vi "Measure IV DC.vi"(0 "dI or Imin":dbl=1e-06, 1 "Imax":dbl=1e-05, 2 "IV Sampling":enum16{"Linear", "Logartihmic"}(ring)=enum."Logartihmic", 3 "IV Type":T1(ring), 4 "6221 Address":string="12", 5 "Ipts":i32=31, 6 "Period (s)":string="0.5", 8 "2182A Address":string="8", 9 "2182A Buffer":string="11") -> (7 "Data array":dbl[][](array[numeric])=[[3e-06, 4.3047886363637716e-07, 1.5313515229084694e-08, 0.14349295454545904, 0.005104505076361564], [3.141e-06, 4.451970222646495e-07, 1.6482457125202314e-08, 0.14173735188304665, 0.005247518982872433], [3.288e-06, 4.509710933322839e-07, 2.1111679012790933e-08, 0.13715665855604742, 0.006420826950362206], [3.442e-06, 4.68688173379921e-07, 1.7706994792785522e-08, 0.136167394938966, 0.005144391282041116], [3.603e-06, 4.984350637099025e-07, 1.7680289772848306e-08, 0.13833890194557383, 0.004907102351609299], [3.772e-06, 5.251681368726084e-07, 2.1467663960858997e-08, 0.1392280320447, 0.005691321304575556], [3.949e-06, 5.275954224918868e-07, 1.1682564654597293e-08, 0.13360228475357985, 0.002958360256925119], [4.134e-06, 5.748183520129533e-07, 1.682018898207155e-08, 0.13904652927260602, 0.004068744311096166], [4.328e-06, 6.067757953443141e-07, 2.4132014421245018e-08, 0.1401977345989635, 0.005575788914335725], [4.531e-06, 6.208427140441133e-07, 2.1984855414698184e-08, 0.13702112426486718, 0.004852097862436147], [4.744e-06, 6.53840833567312e-07, 1.8213175774497554e-08, 0.1378247962831602, 0.0038392023133426547], [4.966e-06, 6.972885085498247e-07, 1.2757960522883814e-08, 0.14041250675590508, 0.0025690617243020165], [5.199e-06, 7.373899562843383e-07, 1.8464251029463237e-08, 0.1418330364078358, 0.003551500486528801], [5.443e-06, 7.869491881659043e-07, 2.1658645151036676e-08, 0.14458004559358886, 0.0039791741964057825], [5.698e-06, 8.296971125303819e-07, 2.6760166214436293e-08, 0.14561198886107088, 0.004696413867047436], [5.965e-06, 8.769758274541976e-07, 1.618644186342838e-08, 0.147020256069438, 0.0027135694657884966], [6.245e-06, 9.014262408876311e-07, 1.6360553186388587e-08, 0.14434367348080562, 0.0026197843372920073], [6.537e-06, 9.540709106298745e-07, 6.51123628419529e-09, 0.1459493514807824, 0.0009960587860173306], [6.844e-06, 9.83842449902655e-07, 2.1788031573785793e-08, 0.14375254966432716, 0.0031835230236390696], [7.165e-06, 1.0389678276192175e-06, 1.6974003144092472e-08, 0.14500597733694592, 0.00236901648905687], [7.501e-06, 1.0842385707281058e-06, 1.7358394306252265e-08, 0.1445458699810833, 0.002314144021630751], [7.852e-06, 1.133576332443823e-06, 2.5546159944328773e-08, 0.14436784671979405, 0.0032534589842497163], [8.221e-06, 1.1828825836341094e-06, 2.5139338002287402e-08, 0.14388548639266627, 0.0030579416132207036], [8.606e-06, 1.2298374260108544e-06, 2.3631436253352804e-08, 0.14290465094246507, 0.002745925662718197], [9.009e-06, 1.316429879745037e-06, 2.1479730496761806e-08, 0.14612386277556189, 0.00238425246939303], [9.432e-06, 1.3727473526086722e-06, 1.6611977521761823e-08, 0.14554149200685668, 0.0017612359543852654], [9.874e-06, 1.440120416246957e-06, 1.667890150606247e-08, 0.1458497484552316, 0.0016891737397268045], [1.0337e-05, 1.4833079536573893e-06, 2.558120171970024e-08, 0.14349501341369733, 0.002474722039247387], [1.0822e-05, 1.552698820767039e-06, 1.7381109531494778e-08, 0.14347614311282933, 0.0016060903281736071], [1.1329e-05, 1.625415578548681e-06, 1.746370239359197e-08, 0.14347387929637928, 0.0015415043157906232], [1.186e-05, 1.7084207500312594e-06, 2.1510520309515023e-08, 0.1440489671189932, 0.0018137032301446057], [1.2416e-05, 1.7752295908882855e-06, 1.866622301771358e-08, 0.14297918741046114, 0.001503400694081313], [1.2998e-05, 1.8543913473684005e-06, 2.184911828979089e-08, 0.14266743709558397, 0.0016809600161402439], [1.3608e-05, 1.9194233726401615e-06, 2.432538101843289e-08, 0.1410511002821988, 0.0017875794399201124], [1.4246e-05, 2.004528849673536e-06, 1.642871958280506e-08, 0.14070818824045597, 0.001153216312144115], [1.4914e-05, 2.1149393689095325e-06, 2.049443802084905e-08, 0.14180899617202175, 0.0013741744683417629], [1.5613e-05, 2.2048839061364533e-06, 2.6366973762175795e-08, 0.1412210277420389, 0.0016887833063585342], [1.6345e-05, 2.299442544196895e-06, 2.4227330364434726e-08, 0.1406817096480205, 0.0014822471926849022], [1.7111e-05, 2.415440098271509e-06, 2.4366737884075522e-08, 0.1411630003080772, 0.001424039383091317], [1.7914e-05, 2.524075530215886e-06, 2.826235852574557e-08, 0.14089960534865947, 0.001577668780046085], [1.8753e-05, 2.649793418562226e-06, 1.806602988302559e-08, 0.14129970770341949, 0.0009633674549685698], [1.9633e-05, 2.777555497862733e-06, 1.9031456611346844e-08, 0.14147381948060575, 0.0009693605975320554], [2.0553e-05, 2.9073259128042663e-06, 1.884648667183435e-08, 0.14145506314427414, 0.0009169701100488663], [2.1517e-05, 3.01009900374514e-06, 1.7512218724119184e-08, 0.13989399097202862, 0.0008138782694668952], [2.2526e-05, 3.160053215899305e-06, 2.1388694840911432e-08, 0.14028470282781252, 0.0009495114463691481], [2.3582e-05, 3.2978086632925506e-06, 2.184497068877449e-08, 0.13984431614335302, 0.0009263408824007502], [2.4687e-05, 3.4422688886650723e-06, 1.9324922599488052e-08, 0.13943650053327955, 0.0007827975290431423], [2.5845e-05, 3.600770279715974e-06, 2.1454878390334967e-08, 0.13932173649510443, 0.000830136521196942], [2.7056e-05, 3.78881652021074e-06, 2.6607076592041645e-08, 0.14003609255657673, 0.0009834076209358975], [2.8325e-05, 3.959486400941646e-06, 2.0862877075484172e-08, 0.13978769288408283, 0.0007365534713321861], [2.9653e-05, 4.17532703440116e-06, 2.3495754463244276e-08, 0.14080622649988736, 0.0007923567417544356], [3.1043e-05, 4.363664112839576e-06, 2.1355539918027872e-08, 0.14056837653704785, 0.00068793415320774], [3.2499e-05, 4.565058439581727e-06, 2.8015991032708503e-08, 0.14046765868432035, 0.0008620570181454353], [3.4023e-05, 4.7549412581003e-06, 2.443505404219635e-08, 0.13975667219528848, 0.0007181922241482629], [3.5618e-05, 4.987050296574805e-06, 1.9740604892462154e-08, 0.1400148884433378, 0.0005542311441535784], [3.7288e-05, 5.248996848807335e-06, 3.229313460677829e-08, 0.14076906374188303, 0.0008660463046228892], [3.9036e-05, 5.512797242351469e-06, 2.5164798391517365e-08, 0.14122341536918406, 0.0006446561735709951], [4.0866e-05, 5.775482443930134e-06, 2.5641849608176923e-08, 0.1413273245223446, 0.0006274616945181061], [4.2782e-05, 6.0405987288507725e-06, 1.9151097766145253e-08, 0.1411948653370757, 0.00044764381670200676], [4.4788e-05, 6.3309968379260555e-06, 2.226396665998493e-08, 0.1413547565849347, 0.0004970966924172754], [4.6888e-05, 6.625184069244457e-06, 3.3556500197253995e-08, 0.14129807347817047, 0.0007156735240840726], [4.9086e-05, 6.952019006582743e-06, 2.894434069415916e-08, 0.14162936492243702, 0.0005896659066568709], [5.1387e-05, 7.288042561715788e-06, 3.348238378409694e-08, 0.14182658185369426, 0.0006515730395644217], [5.3797e-05, 7.650843163495064e-06, 4.295870622361934e-08, 0.14221691104513381, 0.0007985334911541413], [5.6319e-05, 8.029530359919404e-06, 3.787768783183094e-08, 0.14257231768886883, 0.0006725561148427873], [5.896e-05, 8.411537190961149e-06, 3.588480477149981e-08, 0.14266514910042655, 0.0006086296603035924], [6.1724e-05, 8.816997123246386e-06, 4.1323845634023504e-08, 0.14284552399790013, 0.0006694939672416484], [6.4618e-05, 9.252996924901479e-06, 2.9598595842858586e-08, 0.14319534688324428, 0.0004580549667717755], [6.7647e-05, 9.726133083514764e-06, 6.354616463109044e-08, 0.14377774451956132, 0.0009393789027021219], [7.0819e-05, 1.0171226654104171e-05, 2.4735429811748093e-08, 0.14362285056417304, 0.0003492767451072183], [7.4139e-05, 1.0733877514461845e-05, 2.553373296049051e-08, 0.14478044638397936, 0.00034440352527671683], [7.7615e-05, 1.1272707367916842e-05, 3.785521497216293e-08, 0.14523877301960758, 0.0004877306573750297], [8.1254e-05, 1.1873621776794473e-05, 5.281513040074092e-08, 0.14612968932968803, 0.0006500003741445457], [8.5064e-05, 1.2483718740590531e-05, 5.2611155735638645e-08, 0.1467567800784178, 0.0006184890874593088], [8.9052e-05, 1.3137543120825948e-05, 5.422691673347627e-08, 0.14752664870891108, 0.00060893541676185], [9.3227e-05, 1.386324379852252e-05, 5.440153662832007e-08, 0.1487041715224401, 0.000583538423721884], [9.7598e-05, 1.4592835245281601e-05, 4.026019591612147e-08, 0.14951981849301832, 0.0004125104604205155], [0.000102174, 1.5381084091995798e-05, 5.398714968184118e-08, 0.1505381417189872, 0.000528384419537663], [0.000106965, 1.6288471088931045e-05, 5.8580991496088557e-08, 0.15227851249409663, 0.0005476650446042028], [0.00011198, 1.7226805678510595e-05, 4.938284161551474e-08, 0.1538382361002911, 0.0004409969781703406], [0.00011723, 1.8195690188901986e-05, 8.422935795560593e-08, 0.1552135988134606, 0.0007184966131161472], [0.000122726, 1.9440666602087193e-05, 4.754013298598356e-07, 0.1584070743125922, 0.003873680637027489], [0.00012848, 2.046516097520856e-05, 7.72151635638954e-08, 0.15928674482572044, 0.0006009897537663093], [0.000134504, 2.1783101356090124e-05, 6.206822937093433e-08, 0.16195132751509342, 0.00046146010059875043], [0.00014081, 2.3186551308853717e-05, 6.909433376080896e-08, 0.16466551600634696, 0.0004906919519977911], [0.000147412, 2.4779199580014395e-05, 1.0145495447783537e-07, 0.1680948605270561, 0.000688240811316822], [0.000154324, 2.652754000838863e-05, 1.1552426768280052e-07, 0.17189510386193094, 0.0007485826422513706], [0.000161559, 2.8559074860751355e-05, 1.5325269701068354e-07, 0.17677179767608958, 0.000948586565964654], [0.000169134, 3.077335985603851e-05, 1.0749987858342273e-07, 0.1819466213537107, 0.0006355899971822503], [0.000177064, 3.3499875105511105e-05, 1.650934863194129e-07, 0.1891964210992133, 0.0009323944241596987], [0.000185365, 3.675271060014896e-05, 2.140875156213152e-07, 0.19827211501712275, 0.0011549511268109686], [0.000194056, 4.0755061588877246e-05, 2.4656490232316033e-07, 0.21001701358822839, 0.0012705863375683326], [0.000203154, 4.5583701866592996e-05, 2.88002297844996e-07, 0.22438003616267954, 0.0014176550687901592], [0.000212679, 4.6885277578993986e-05, 1.8559705682216518e-07, 0.22045090290528913, 0.0008726628243604925], [0.000222651, 5.437543406576834e-05, 3.339108756556848e-07, 0.24421823421304345, 0.0014997052591530459], [0.00023309, 6.52378590218662e-05, 4.087905596822482e-07, 0.27988270205442617, 0.001753788492351659], [0.000244018, 8.078607685365366e-05, 5.535103789648243e-07, 0.33106605600264594, 0.0022683178247704036], [0.000255459, 0.00010528381597780848, 7.381396785359974e-07, 0.4121358651596087, 0.0028894643701572365], [0.000267436, 0.00014543789662409701, 1.3105807197850573e-06, 0.5438231824589697, 0.004900539642325855], [0.000279975, 0.0002164796371265307, 1.9276740217917436e-06, 0.7732105978267013, 0.006885164824687003], [0.000293101, 0.0003364904621252049, 1.684747078560466e-06, 1.1480358720209243, 0.005748008633749002], [0.000306843, 0.0005085274541554971, 1.1729721508444118e-06, 1.6572887572976966, 0.003822711128637159], [0.00032123, 0.0006778030568942108, 6.876202556105575e-07, 2.1100241474775423, 0.002140585423561179], [0.000336291, 0.0008259884419767413, 4.1136515560515926e-07, 2.456171714309159, 0.0012232416437108315], [0.000352057, 0.0009578186150472369, 1.982003546971834e-07, 2.7206350535488197, 0.0005629780254253811], [0.000368564, 0.0010792919557635811, 2.0647815388337988e-07, 2.928370529307206, 0.000560223336743089], [0.000385844, 0.0011932501573751963, 1.6637910902181772e-07, 3.092571498779808, 0.00043120823188080604], [0.000403934, 0.0013019248018429324, 6.616749526058568e-08, 3.2231126912885086, 0.00016380768952498596], [0.000422872, 0.0014063865904152633, 5.9536173907995785e-08, 3.3257973817497097, 0.00014079005918574836], [0.000442699, 0.0015057233089116322, 5.663047245823841e-08, 3.40123494498888, 0.00012792094054479096], [0.000463455, 0.001602269073650902, 2.8720907727946024e-08, 3.457226858380861, 6.197129759727703e-05], [0.000485184, 0.0016952998337987934, 2.339000992951633e-08, 3.494137963739104, 4.820853517328752e-05], [0.000507932, 0.001786953980172823, 1.5693892498723275e-08, 3.5180968715749805, 3.089762507328397e-05], [0.000531746, 0.001878406864318594, 1.5599137248114433e-08, 3.5325265527499856, 2.9335692695599837e-05], [0.000556677, 0.0019710559814260058, 1.0823648816328349e-08, 3.5407534017500377, 1.94433195844778e-05], [0.000582777, 0.002065715042834221, 1.3096483346757564e-08, 3.5446063294093983, 2.2472546697549086e-05], [0.0006101, 0.002163659391303364, 1.0976700998578674e-08, 3.546401231442983, 1.7991642351382843e-05], [0.000638705, 0.0022654655576607543, 1.1177311405105967e-08, 3.5469669998837556, 1.749995914405863e-05], [0.00066865, 0.0023721142447375295, 1.5030529513429894e-08, 3.5476172059186863, 2.2478919484677922e-05], [0.0007, 0.002483311050336363, 1.5199603028809162e-08, 3.547587214766233, 2.1713718612584518e-05]])   [LabVIEW 2020]
uses:
  <vilib>/Analysis/1siggen.llb/Ramp Pattern by Delta.vi
  <vilib>/Analysis/NI_AALBase.lvlib
panel:
  in  "Correct Voltage Offset":bool=TRUE
  out "Voltage Offset":dbl=2.1003043299999988e-05
  in  "Debug Mode":bool
  out "Resistance STD":dbl=2.1713718612584518e-05
  out "Resistance":dbl=3.5475872147662333
  in  "NPLC":string="1"
  in  "2182A Range":string="0.01"
  out "I-V Plot":cluster{"Ramp Pattern":dbl[], dbl[]}[](graph)=[{"Ramp Pattern"=[3e-06, 3.141e-06, 3.288e-06, 3.442e-06, 3.603e-06, 3.772e-06, 3.949e-06, 4.134e-06, 4.328e-06, 4.531e-06, 4.744e-06, 4.966e-06, 5.199e-06, 5.443e-06, 5.698e-06, 5.965e-06, 6.245e-06, 6.537e-06, 6.844e-06, 7.165e-06, 7.501e-06, 7.852e-06, 8.221e-06, 8.606e-06, 9.009e-06, 9.432e-06, 9.874e-06, 1.0337e-05, 1.0822e-05, 1.1329e-05, 1.186e-05, 1.2416e-05, 1.2998e-05, 1.3608e-05, 1.4246e-05, 1.4914e-05, 1.5613e-05, 1.6345e-05, 1.7111e-05, 1.7914e-05, 1.8753e-05, 1.9633e-05, 2.0553e-05, 2.1517e-05, 2.2526e-05, 2.3582e-05, 2.4687e-05, 2.5845e-05, 2.7056e-05, 2.8325e-05, 2.9653e-05, 3.1043e-05, 3.2499e-05, 3.4023e-05, 3.5618e-05, 3.7288e-05, 3.9036e-05, 4.0866e-05, 4.2782e-05, 4.4788e-05, 4.6888e-05, 4.9086e-05, 5.1387e-05, 5.3797e-05, 5.6319e-05, 5.896e-05, 6.1724e-05, 6.4618e-05, 6.7647e-05, 7.0819e-05, 7.4139e-05, 7.7615e-05, 8.1254e-05, 8.5064e-05, 8.9052e-05, 9.3227e-05, 9.7598e-05, 0.000102174, 0.000106965, 0.00011198, 0.00011723, 0.000122726, 0.00012848, 0.000134504, 0.00014081, 0.000147412, 0.000154324, 0.000161559, 0.000169134, 0.000177064, 0.000185365, 0.000194056, 0.000203154, 0.000212679, 0.000222651, 0.00023309, 0.000244018, 0.000255459, 0.000267436, 0.000279975, 0.000293101, 0.000306843, 0.00032123, 0.000336291, 0.000352057, 0.000368564, 0.000385844, 0.000403934, 0.000422872, 0.000442699, 0.000463455, 0.000485184, 0.000507932, 0.000531746, 0.000556677, 0.000582777, 0.0006101, 0.000638705, 0.00066865, 0.0007], [4.3047886363637716e-07, 4.451970222646495e-07, 4.509710933322839e-07, 4.68688173379921e-07, 4.984350637099025e-07, 5.251681368726084e-07, 5.275954224918868e-07, 5.748183520129533e-07, 6.067757953443141e-07, 6.208427140441133e-07, 6.53840833567312e-07, 6.972885085498247e-07, 7.373899562843383e-07, 7.869491881659043e-07, 8.296971125303819e-07, 8.769758274541976e-07, 9.014262408876311e-07, 9.540709106298745e-07, 9.83842449902655e-07, 1.0389678276192175e-06, 1.0842385707281058e-06, 1.133576332443823e-06, 1.1828825836341094e-06, 1.2298374260108544e-06, 1.316429879745037e-06, 1.3727473526086722e-06, 1.440120416246957e-06, 1.4833079536573893e-06, 1.552698820767039e-06, 1.625415578548681e-06, 1.7084207500312594e-06, 1.7752295908882855e-06, 1.8543913473684005e-06, 1.9194233726401615e-06, 2.004528849673536e-06, 2.1149393689095325e-06, 2.2048839061364533e-06, 2.299442544196895e-06, 2.415440098271509e-06, 2.524075530215886e-06, 2.649793418562226e-06, 2.777555497862733e-06, 2.9073259128042663e-06, 3.01009900374514e-06, 3.160053215899305e-06, 3.2978086632925506e-06, 3.4422688886650723e-06, 3.600770279715974e-06, 3.78881652021074e-06, 3.959486400941646e-06, 4.17532703440116e-06, 4.363664112839576e-06, 4.565058439581727e-06, 4.7549412581003e-06, 4.987050296574805e-06, 5.248996848807335e-06, 5.512797242351469e-06, 5.775482443930134e-06, 6.0405987288507725e-06, 6.3309968379260555e-06, 6.625184069244457e-06, 6.952019006582743e-06, 7.288042561715788e-06, 7.650843163495064e-06, 8.029530359919404e-06, 8.411537190961149e-06, 8.816997123246386e-06, 9.252996924901479e-06, 9.726133083514764e-06, 1.0171226654104171e-05, 1.0733877514461845e-05, 1.1272707367916842e-05, 1.1873621776794473e-05, 1.2483718740590531e-05, 1.3137543120825948e-05, 1.386324379852252e-05, 1.4592835245281601e-05, 1.5381084091995798e-05, 1.6288471088931045e-05, 1.7226805678510595e-05, 1.8195690188901986e-05, 1.9440666602087193e-05, 2.046516097520856e-05, 2.1783101356090124e-05, 2.3186551308853717e-05, 2.4779199580014395e-05, 2.652754000838863e-05, 2.8559074860751355e-05, 3.077335985603851e-05, 3.3499875105511105e-05, 3.675271060014896e-05, 4.0755061588877246e-05, 4.5583701866592996e-05, 4.6885277578993986e-05, 5.437543406576834e-05, 6.52378590218662e-05, 8.078607685365366e-05, 0.00010528381597780848, 0.00014543789662409701, 0.0002164796371265307, 0.0003364904621252049, 0.0005085274541554971, 0.0006778030568942108, 0.0008259884419767413, 0.0009578186150472369, 0.0010792919557635811, 0.0011932501573751963, 0.0013019248018429324, 0.0014063865904152633, 0.0015057233089116322, 0.001602269073650902, 0.0016952998337987934, 0.001786953980172823, 0.001878406864318594, 0.0019710559814260058, 0.002065715042834221, 0.002163659391303364, 0.0022654655576607543, 0.0023721142447375295, 0.002483311050336363]}, {"Ramp Pattern"=[3e-06, 3.141e-06, 3.288e-06, 3.442e-06, 3.603e-06, 3.772e-06, 3.949e-06, 4.134e-06, 4.328e-06, 4.531e-06, 4.744e-06, 4.966e-06, 5.199e-06, 5.443e-06, 5.698e-06, 5.965e-06, 6.245e-06, 6.537e-06, 6.844e-06, 7.165e-06, 7.501e-06, 7.852e-06, 8.221e-06, 8.606e-06, 9.009e-06, 9.432e-06, 9.874e-06, 1.0337e-05, 1.0822e-05, 1.1329e-05, 1.186e-05, 1.2416e-05, 1.2998e-05, 1.3608e-05, 1.4246e-05, 1.4914e-05, 1.5613e-05, 1.6345e-05, 1.7111e-05, 1.7914e-05, 1.8753e-05, 1.9633e-05, 2.0553e-05, 2.1517e-05, 2.2526e-05, 2.3582e-05, 2.4687e-05, 2.5845e-05, 2.7056e-05, 2.8325e-05, 2.9653e-05, 3.1043e-05, 3.2499e-05, 3.4023e-05, 3.5618e-05, 3.7288e-05, 3.9036e-05, 4.0866e-05, 4.2782e-05, 4.4788e-05, 4.6888e-05, 4.9086e-05, 5.1387e-05, 5.3797e-05, 5.6319e-05, 5.896e-05, 6.1724e-05, 6.4618e-05, 6.7647e-05, 7.0819e-05, 7.4139e-05, 7.7615e-05, 8.1254e-05, 8.5064e-05, 8.9052e-05, 9.3227e-05, 9.7598e-05, 0.000102174, 0.000106965, 0.00011198, 0.00011723, 0.000122726, 0.00012848, 0.000134504, 0.00014081, 0.000147412, 0.000154324, 0.000161559, 0.000169134, 0.000177064, 0.000185365, 0.000194056, 0.000203154, 0.000212679, 0.000222651, 0.00023309, 0.000244018, 0.000255459, 0.000267436, 0.000279975, 0.000293101, 0.000306843, 0.00032123, 0.000336291, 0.000352057, 0.000368564, 0.000385844, 0.000403934, 0.000422872, 0.000442699, 0.000463455, 0.000485184, 0.000507932, 0.000531746, 0.000556677, 0.000582777, 0.0006101, 0.000638705, 0.00066865, 0.0007], [0.14349295454545904, 0.14173735188304665, 0.13715665855604742, 0.136167394938966, 0.13833890194557383, 0.1392280320447, 0.13360228475357985, 0.13904652927260602, 0.1401977345989635, 0.13702112426486718, 0.1378247962831602, 0.14041250675590508, 0.1418330364078358, 0.14458004559358886, 0.14561198886107088, 0.147020256069438, 0.14434367348080562, 0.1459493514807824, 0.14375254966432716, 0.14500597733694592, 0.1445458699810833, 0.14436784671979405, 0.14388548639266627, 0.14290465094246507, 0.14612386277556189, 0.14554149200685668, 0.1458497484552316, 0.14349501341369733, 0.14347614311282933, 0.14347387929637928, 0.1440489671189932, 0.14297918741046114, 0.14266743709558397, 0.1410511002821988, 0.14070818824045597, 0.14180899617202175, 0.1412210277420389, 0.1406817096480205, 0.1411630003080772, 0.14089960534865947, 0.14129970770341949, 0.14147381948060575, 0.14145506314427414, 0.13989399097202862, 0.14028470282781252, 0.13984431614335302, 0.13943650053327955, 0.13932173649510443, 0.14003609255657673, 0.13978769288408283, 0.14080622649988736, 0.14056837653704785, 0.14046765868432035, 0.13975667219528848, 0.1400148884433378, 0.14076906374188303, 0.14122341536918406, 0.1413273245223446, 0.1411948653370757, 0.1413547565849347, 0.14129807347817047, 0.14162936492243702, 0.14182658185369426, 0.14221691104513381, 0.14257231768886883, 0.14266514910042655, 0.14284552399790013, 0.14319534688324428, 0.14377774451956132, 0.14362285056417304, 0.14478044638397936, 0.14523877301960758, 0.14612968932968803, 0.1467567800784178, 0.14752664870891108, 0.1487041715224401, 0.14951981849301832, 0.1505381417189872, 0.15227851249409663, 0.1538382361002911, 0.1552135988134606, 0.1584070743125922, 0.15928674482572044, 0.16195132751509342, 0.16466551600634696, 0.1680948605270561, 0.17189510386193094, 0.17677179767608958, 0.1819466213537107, 0.1891964210992133, 0.19827211501712275, 0.21001701358822839, 0.22438003616267954, 0.22045090290528913, 0.24421823421304345, 0.27988270205442617, 0.33106605600264594, 0.4121358651596087, 0.5438231824589697, 0.7732105978267013, 1.1480358720209243, 1.6572887572976966, 2.1100241474775423, 2.456171714309159, 2.7206350535488197, 2.928370529307206, 3.092571498779808, 3.2231126912885086, 3.3257973817497097, 3.40123494498888, 3.457226858380861, 3.494137963739104, 3.5180968715749805, 3.5325265527499856, 3.5407534017500377, 3.5446063294093983, 3.546401231442983, 3.5469669998837556, 3.5476172059186863, 3.547587214766233]}]
  out "Votlage STD":dbl=1.5199603028809162e-08
  out "Voltage":dbl=0.002483311050336363
  out "Current Now":string="700.000E-6"
  in  "stop":bool
  in  "Measure?":bool=TRUE
  out "Current Samples":dbl[](array[numeric])=[3e-06, 3.1406549088857057e-06, 3.2879044189026255e-06, 3.442057717724511e-06, 3.603438489279804e-06, 3.772385593408102e-06, 3.9492537773822905e-06, 4.134414420790367e-06, 4.32825631534104e-06, 4.531186481230464e-06, 4.743631021784333e-06, 4.966036018169827e-06, 5.198868466056096e-06, 5.442617256190057e-06, 5.697794200946451e-06, 5.9649351090076585e-06, 6.244600910429864e-06, 6.537378834457898e-06, 6.8438836425619034e-06, 7.164758919284874e-06, 7.50067842361156e-06, 7.852347503696246e-06, 8.220504577920009e-06, 8.605922685387296e-06, 9.009411109117489e-06, 9.431817075339749e-06, 9.874027532459264e-06, 1.0336971013430267e-05, 1.0821619585446334e-05, 1.1328990891041906e-05, 1.1860150284890736e-05, 1.2416213070788092e-05, 1.2998346843513827e-05, 1.3607773940493573e-05, 1.4245774008406035e-05, 1.4913686690125602e-05, 1.5612914437642126e-05, 1.6344925456864413e-05, 1.711125679049072e-05, 1.791351754541951e-05, 1.875339227147733e-05, 1.9632644498558175e-05, 2.0553120439601558e-05, 2.151675286718458e-05, 2.2525565171867943e-05, 2.358167561081731e-05, 2.468730175562123e-05, 2.5844765148644834e-05, 2.7056496177696535e-05, 2.8325039179243306e-05, 2.9653057780890138e-05, 3.1043340494341355e-05, 3.249880657058786e-05, 3.402251212961459e-05, 3.561765657749918e-05, 3.728758932437601e-05, 3.9035816817371893e-05, 4.0866009903280735e-05, 4.2782011536436836e-05, 4.4787844847971736e-05, 4.688772159339793e-05, 4.908605099625717e-05, 5.138744900640303e-05, 5.379674799235784e-05, 5.631900688809529e-05, 5.895952181555477e-05, 6.172383720519199e-05, 6.461775743791608e-05, 6.764735903285898e-05, 7.081900340656744e-05, 7.413935023040985e-05, 7.761537141424442e-05, 8.125436574571134e-05, 8.506397421588756e-05, 8.905219606348478e-05, 9.32274055712786e-05, 9.759836965003821e-05, 0.00010217426624687807, 0.0001069647036166842, 0.00011197974049708122, 0.00011722990722930185, 0.00012272622786930757, 0.00012848024333558884, 0.000134504035642249, 0.00014081025326825573, 0.0001474121377161289, 0.00015432355131583193, 0.00016155900633224755, 0.00016913369543735668, 0.00017706352361110468, 0.00018536514153793865, 0.0001940559805691401, 0.00020315428932436634, 0.00021267917200925264, 0.00022265062852953554, 0.0002330895964859245, 0.00024401799513790236, 0.00025545877142876697, 0.0002674359481685561, 0.0002799746744760263, 0.00029310127858560314, 0.0003068433231301837, 0.0003212296630158713, 0.00033629050601016584, 0.0003520574761708282, 0.0003685636802486078, 0.00038584377720325734, 0.00040393405097880397, 0.0004228724866908901, 0.00044269885038614946, 0.0004634547725411065, 0.0004851838354759112, 0.0005079316648664714, 0.0005317460255471244, 0.000556676921805013, 0.0005827767023767664, 0.0006101001703679381, 0.0006387046983260229, 0.0006686503487086629, 0.0006999999999999999]
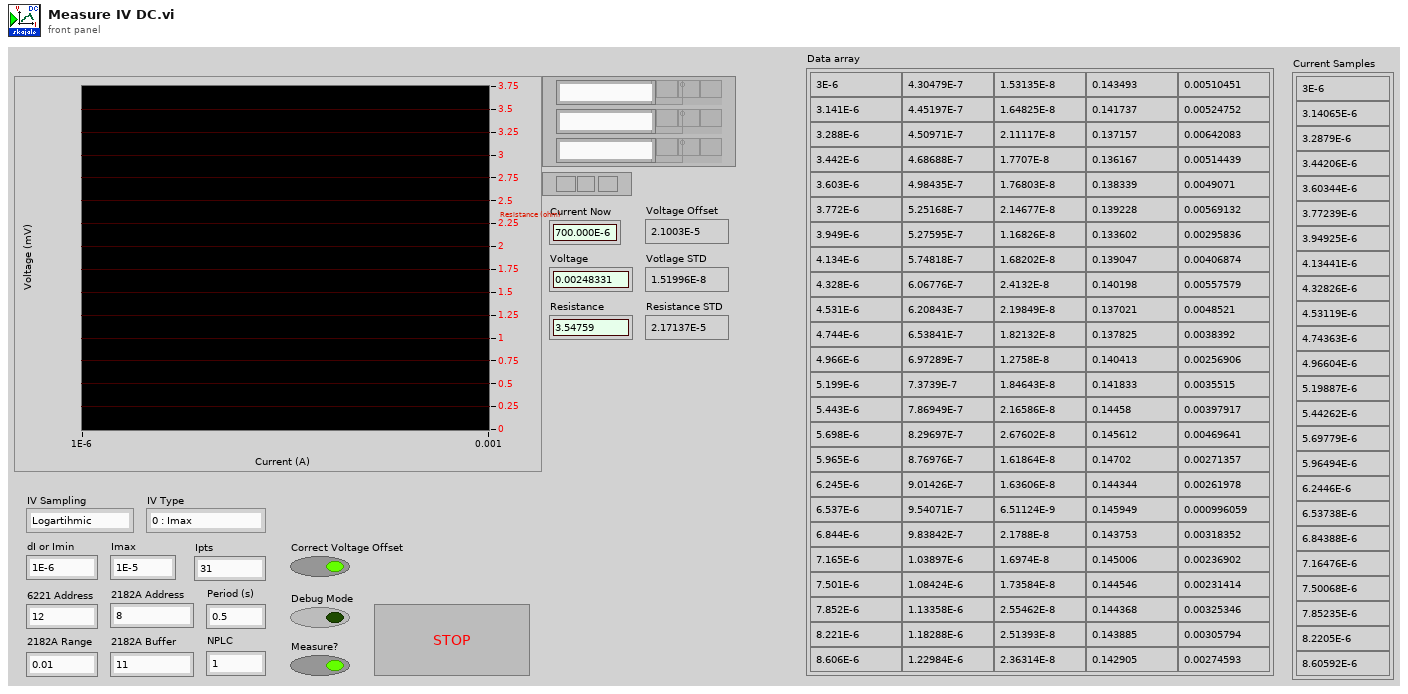
[diagram p1: front panel]
types:
  T1 = enum16{"0 : Imax", "0 : Imax : 0", "0 : Imax : -Imax : 0", "-Imax : 0 : Imax"}
  T2 = cluster{"Data array":dbl[], "Data array":dbl[]}[]
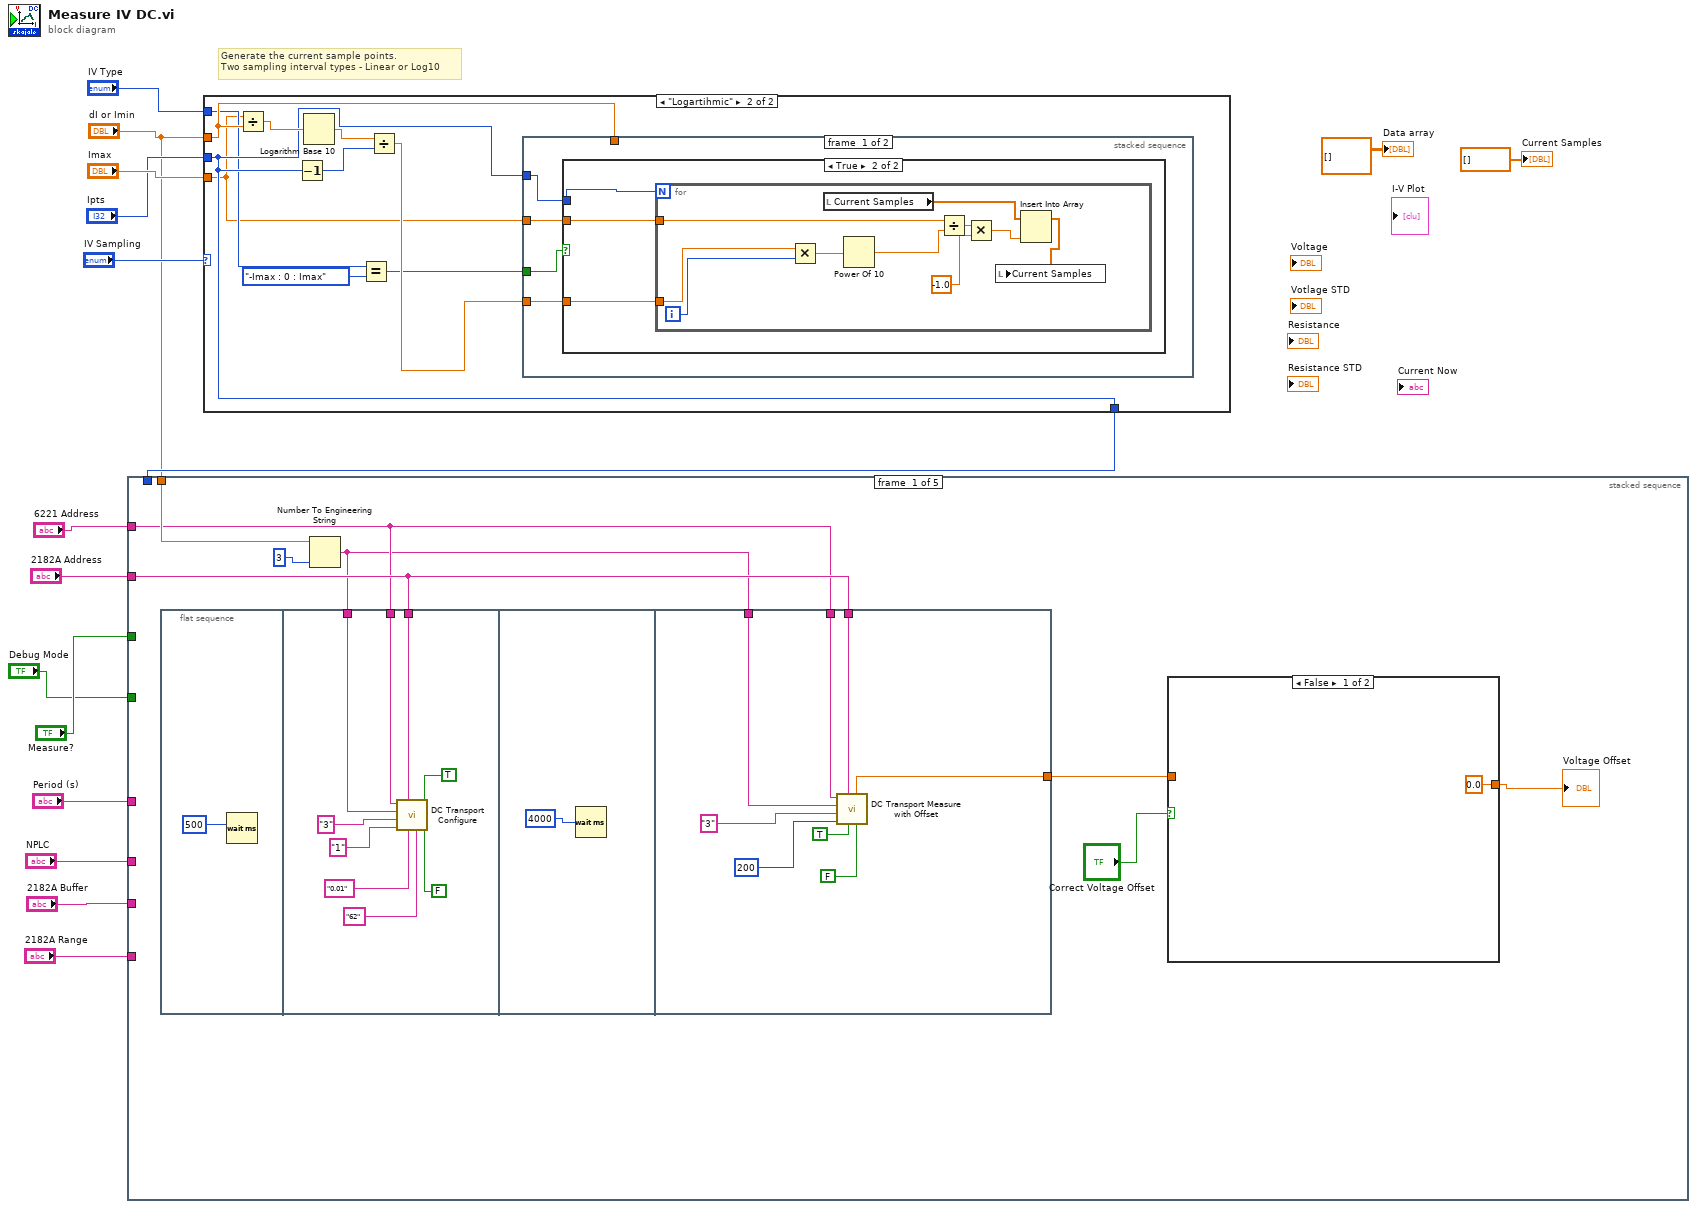
[diagram p0: block diagram]
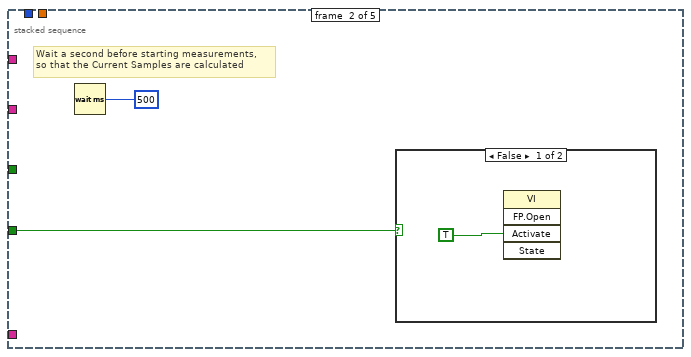
[diagram p3: hidden frame]
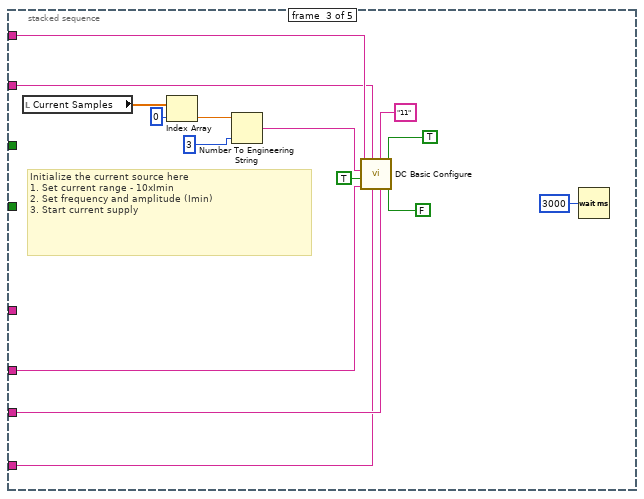
[diagram p5: hidden frame]
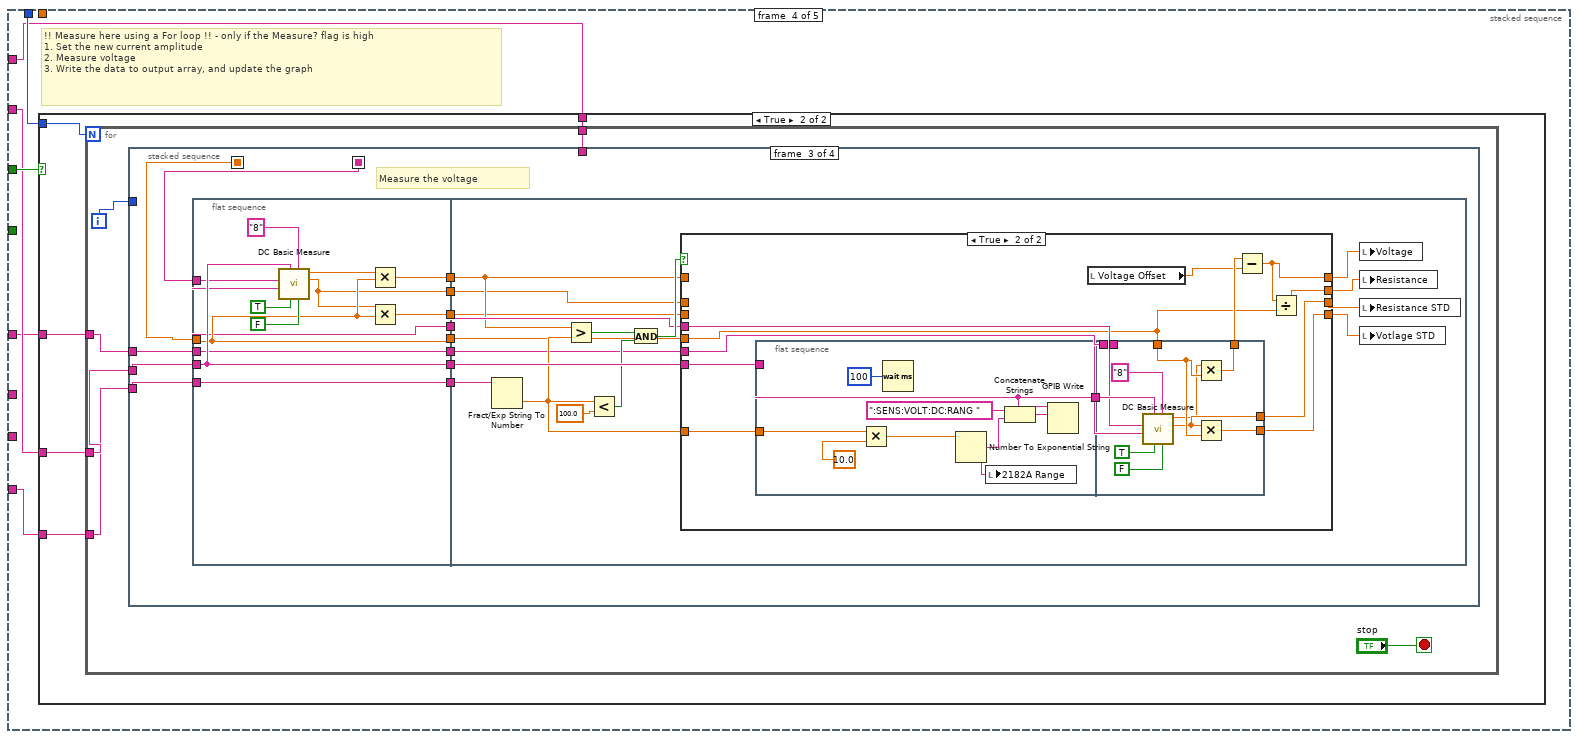
[diagram p6: hidden frame]
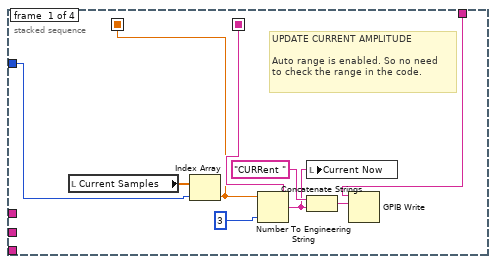
[diagram p8: hidden frame]
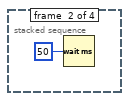
[diagram p9: hidden frame]
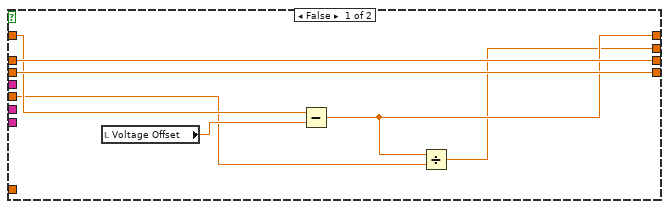
[diagram p10: hidden frame]
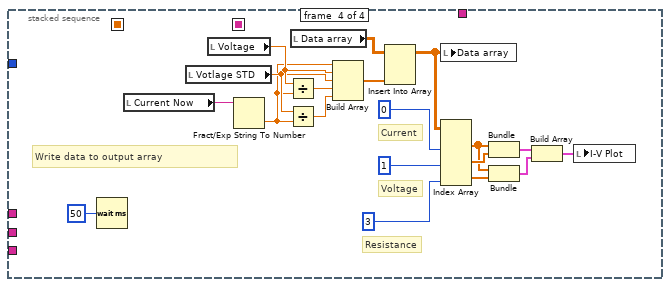
[diagram p11: hidden frame]
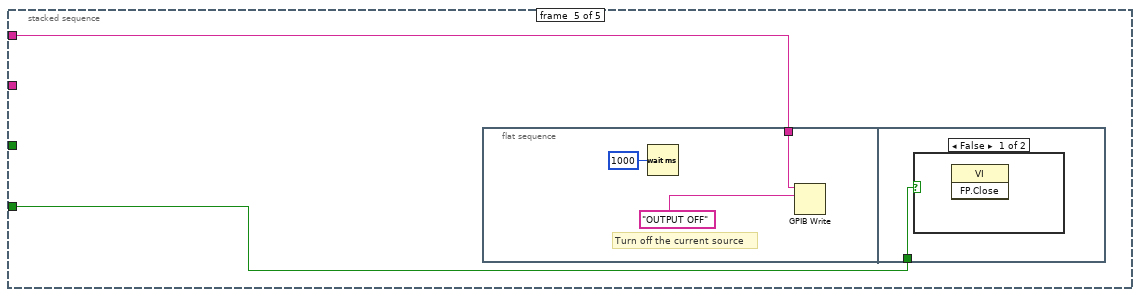
[diagram p12: hidden frame]
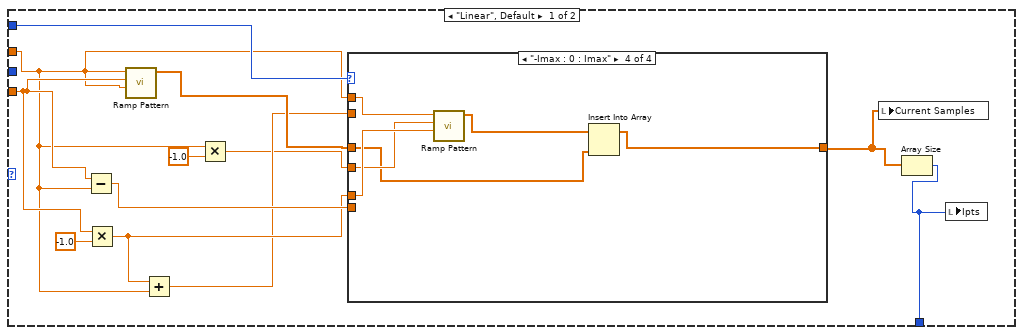
[diagram p14: hidden frame]
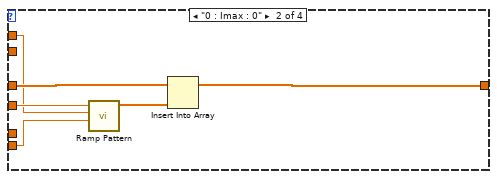
[diagram p16: hidden frame]
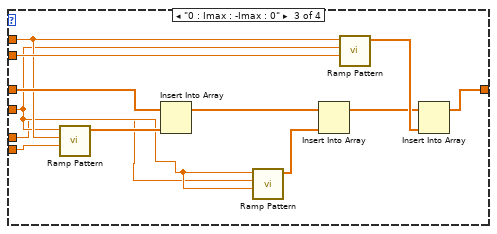
[diagram p17: hidden frame]
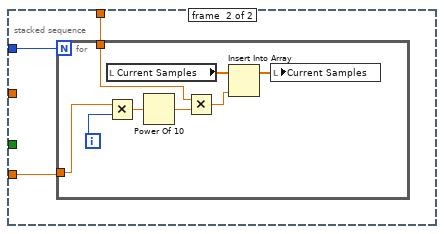
[diagram p19: hidden frame]
diagram:
  # "Generate the current sample points.\nTwo sampling interval types - Linear or Log10"
  n1 = case shown="\"Logartihmic\"" "IV Sampling" {
    tunnel: "Ipts" -> [_ w58]
    tunnel: "Imax" -> [w24 w54]
    tunnel: "dI or Imin" -> [w18 w59]
    tunnel: "IV Type" -> [w28 w57]
    tunnel: [w17 w58] -> w2
    frame "Linear", Default {
      n2 = Subtract(x=w24, y=w18) -> (x-y=w26:dbl)
      n3 = Multiply(x=w24, y=-1.0) -> (x*y=w23:dbl)
      n4 = call-poly <vilib>:"Ramp Pattern.vi"("start"=w18, "end"=w24, "delta"=w18) -> ("Ramp Pattern"=w27:dbl[])  [unwired: 6 in, 2 out]
      n5 = Add(x=w23, y=w18) -> (x+y=w22:dbl)
      n6 = Multiply(x=w18, y=-1.0) -> (x*y=w20:dbl)
      n7 = case shown="\"-Imax : 0 : Imax\"" w28 {
        tunnel: w27 -> [w29 w34 w46 w49]
        tunnel: [w29 w32 w44 w48] -> w19
        tunnel: w26 -> [_ w35 w47 _]
        tunnel: w18 -> [_ w30 w41 w53]
        tunnel: w23 -> [_ _ w39 w52]
        tunnel: w22 -> [_ _ w43 _]
        tunnel: w20 -> [_ w31 w40 w51]
        frame "0 : Imax", Default {
          # "For Linear sampling, possible to choose sweep type\n- Forward, 0:Imax\n-Half cycle, 0:Imax:0\n- Full cycles, 0:Imax:-Imax:0"
          # "Pass on the 0:Imax samples are they are"
        }
        frame "0 : Imax : 0" {
          n8 = call-poly <vilib>:"Ramp Pattern.vi"("start"=w35, "end"=w30, "delta"=w31) -> ("Ramp Pattern"=w33:dbl[])  [unwired: 6 in, 2 out]
          n9 = Insert Into Array(array=w34, new element=w33) -> (w32:dbl[])  [unwired: 1 in]
        }
        frame "0 : Imax : -Imax : 0" {
          n10 = call-poly <vilib>:"Ramp Pattern.vi"("start"=w47, "end"=w41, "delta"=w40) -> ("Ramp Pattern"=w45:dbl[])  [unwired: 6 in, 2 out]
          n11 = Insert Into Array(array=w46, new element=w45) -> (w38:dbl[])  [unwired: 1 in]
          n12 = call-poly <vilib>:"Ramp Pattern.vi"("start"=w40, "end"=w39, "delta"=w40) -> ("Ramp Pattern"=w36:dbl[])  [unwired: 6 in, 2 out]
          n13 = Insert Into Array(array=w38, new element=w36) -> (w37:dbl[])  [unwired: 1 in]
          n14 = call-poly <vilib>:"Ramp Pattern.vi"("start"=w43, "end"=w40, "delta"=w41) -> ("Ramp Pattern"=w42:dbl[])  [unwired: 6 in, 2 out]
          n15 = Insert Into Array(array=w37, new element=w42) -> (w44:dbl[])  [unwired: 1 in]
        }
        frame "-Imax : 0 : Imax" {
          n16 = call-poly <vilib>:"Ramp Pattern.vi"("start"=w52, "end"=w51, "delta"=w53) -> ("Ramp Pattern"=w50:dbl[])  [unwired: 6 in, 2 out]
          n17 = Insert Into Array(array=w50, new element=w49) -> (w48:dbl[])  [unwired: 1 in]
        }
      }
      n18 = local write "Current Samples"(w19) -> ()
      n19 = Array Size(array=w19) -> (size(s)=w17:i32)
      n20 = local write "Ipts"(w17) -> ()
    }
    frame "Logartihmic" {
      n21 = Divide(x=w54, y=w59) -> (x/y=w63:dbl)
      n22 = Decrement(x=w58) -> (x-1=w61:i32)
      n23 = Logarithm Base 10(1:w63) -> (0:w62:dbl)
      n24 = Equal?(x=w57, y=T1."-Imax : 0 : Imax") -> (x = y?=w55:bool)
      n25 = Divide(x=w62, y=w61) -> (x/y=w60:dbl)
      n26 = stacked-sequence {
        tunnel: w60 -> [w66 w82]
        tunnel: w58 -> [w67 w81]
        tunnel: w59 -> [_ w83]
        tunnel: w55 -> [w65 _]
        tunnel: w54 -> [w64 _]
        frame #0 {
          n27 = case shown="True" w65 {
            tunnel: w67 -> [_ w70]
            tunnel: w66 -> [_ w69]
            tunnel: w64 -> [_ w68]
            frame False {
            }
            frame True {
              n28 = for {
                N: w70 -> [_]
                tunnel: w69 -> [w74]
                tunnel: w68 -> [w71]
                i -> [w80]
                n29 = Multiply(x=w74, y=w80) -> (x*y=w79:dbl)
                n30 = local read "Current Samples"() -> (w72:dbl[])
                n31 = Power Of 10(x=w79) -> (10^x=w77:dbl)
                n32 = Divide(x=w71, y=w77) -> (x/y=w78:dbl)
                n33 = Multiply(x=w78, y=-1.0) -> (x*y=w76:dbl)
                n34 = Insert Into Array(array=w72, new element=w76) -> (w73:dbl[])  [unwired: 1 in]
                n35 = local write "Current Samples"(w73) -> ()
              }
            }
          }
        }
        frame #1 {
          n36 = for {
            N: w81 -> [_]
            tunnel: w82 -> [w89]
            tunnel: w83 -> [w85]
            i -> [w88]
            n37 = local read "Current Samples"() -> (w90:dbl[])
            n38 = Multiply(x=w89, y=w88) -> (x*y=w87:dbl)
            n39 = Power Of 10(x=w87) -> (10^x=w86:dbl)
            n40 = Multiply(x=w85, y=w86) -> (x*y=w84:dbl)
            n41 = Insert Into Array(array=w90, new element=w84) -> (w91:dbl[])  [unwired: 1 in]
            n42 = local write "Current Samples"(w91) -> ()
          }
        }
      }
    }
  }
  n43 = stacked-sequence {
    tunnel: w2 -> [_ _ _ w144 _]
    tunnel: "2182A Buffer" -> [_ _ w133 _ _]
    tunnel: "2182A Range" -> [_ _ w132 w140 _]
    tunnel: "NPLC" -> [_ _ w131 _ _]
    tunnel: "6221 Address" -> [w96 _ w129 w139 w264]
    tunnel: "2182A Address" -> [w97 _ w128 w142 _]
    tunnel: "Measure?" -> [_ _ _ w143 _]
    tunnel: "Period (s)" -> [_ _ _ w141 _]
    tunnel: "Debug Mode" -> [_ w121 _ _ w265]
    tunnel: "dI or Imin" -> [w98 _ _ _ _]
    frame #0 {
      n44 = flat-sequence {
        tunnel: w97 -> [w110]
        tunnel: w96 -> [w109]
        tunnel: w95 -> [w108]
        tunnel: w97 -> [w120]
        tunnel: w96 -> [w119]
        tunnel: w95 -> [w118]
        tunnel: [w113] -> w93
        frame #0 {
          n45 = Wait (ms)(milliseconds to wait=u32 500) -> ()  [unwired: 1 out]
        }
        frame #1 {
          n46 = call "DC Transport Configure.vi"("Channel 2"=FALSE, "Channel 1"=TRUE, "Voltmeter Buffer Size"="62", "Voltmeter Range (V)"="0.01", "Voltmeter 1 Address"=w110, "NPLC"="1", "Time Period (s)"="3", "Current Amplitude"=w108, "6221 Address"=w109) -> ()  [unwired: 3 in]
        }
        frame #2 {
          n47 = Wait (ms)(milliseconds to wait=u32 4000) -> ()  [unwired: 1 out]
        }
        frame #3 {
          n48 = call "DC Transport Measure with Offset.vi"("Channel 2"=FALSE, "Channel 1"=TRUE, "Voltmeter 1 Address"=w120, "tpad"=200, "Period (s)"="3", "Amplitude (A)"=w118, "6221 Address"=w119) -> ("Voltmeter 1 Offset"=w113:dbl)  [unwired: 4 out]
        }
      }
      n49 = Number To Engineering String(2:i16 3 ("precision (6)"), 4:w98) -> (0:w95:string)  [unwired: 2 in]
      n50 = case shown="False" "Correct Voltage Offset" {
        tunnel: w93 -> [_ w101]
        tunnel: [0.0 ("Voltmeter 1 Offset") w101] -> w92
        frame False {
        }
        frame True {
        }
      }
      "Voltage Offset" <- w92
    }
    frame #1 {
      # "Wait a second before starting measurements,\nso that the Current Samples are calculated"
      n51 = Wait (ms)(milliseconds to wait=u32 500) -> ()  [unwired: 1 out]
      n52 = case shown="False" w121 {
        frame False {
          n53 = invoke class="VI" method="FP.Open"("Activate"=TRUE ("Activate?")) -> ()  [unwired: 4 in, 5 out]
        }
        frame True {
        }
      }
    }
    frame #2 {
      # "Initialize the current source here\n1. Set current range - 10xImin\n2. Set frequency and amplitude (Imin)\n3. Start current supply"
      n54 = local read "Current Samples"() -> (w138:dbl[])
      n55 = Index Array(array=w138, index=0) -> (element=w136:dbl)
      n56 = Number To Engineering String(2:i16 3 ("precision (6)"), 4:w136) -> (0:w130:string)  [unwired: 2 in]
      n57 = call "DC Basic Configure.vi"("Channel 2"=FALSE, "Channel 1"=TRUE, "Voltmeter Buffer Size"=w133, "Voltmeter 2 Address"="11", "Voltmeter Range (V)"=w132, "Voltmeter 1 Address"=w128, "NPLC"=w131, "INIT Wave"=TRUE, "Current Amplitude"=w130, "6221 Address"=w129) -> ()  [unwired: 2 in]
      n58 = Wait (ms)(milliseconds to wait=u32 3000) -> ()  [unwired: 1 out]
    }
    frame #3 {
      # "!! Measure here using a For loop !! - only if the Measure? flag is high\n1. Set the new current amplitude\n2. Measure voltage\n3. Write the data to output array, and update the graph"
      n59 = case shown="True" w143 {
        tunnel: w144 -> [_ w149]
        tunnel: w142 -> [_ w148]
        tunnel: w141 -> [_ w147]
        tunnel: w140 -> [_ w146]
        tunnel: w139 -> [_ w145]
        frame False {
        }
        frame True {
          n60 = for {
            N: w149 -> [_]
            tunnel: w148 -> [w153]
            tunnel: w147 -> [w152]
            tunnel: w146 -> [w151]
            tunnel: w145 -> [w150]
            i -> [w154]
            stop <- "stop" stop-if-true
            n61 = stacked-sequence {
              seq-local: [w158 _ _ _] -> [_ _ w176 _]
              seq-local: [w157 _ _ _] -> [_ _ w174 _]
              tunnel: w154 -> [w162 _ _ _]
              tunnel: w153 -> [_ _ w177 _]
              tunnel: w152 -> [_ _ w175 _]
              tunnel: w151 -> [_ _ w171 _]
              tunnel: w150 -> [w156 _ _ _]
              frame #0 {
                # "UPDATE CURRENT AMPLITUDE\n\nAuto range is enabled. So no need \nto check the range in the code."
                n62 = local read "Current Samples"() -> (w163:dbl[])
                n63 = Index Array(array=w163, index=w162) -> (element=w157:dbl)
                n64 = Number To Engineering String(2:i16 3 ("precision (6)"), 4:w157) -> (0:w158:string)  [unwired: 2 in]
                n65 = local write "Current Now"(w158) -> ()
                n66 = Concatenate Strings("CURRent " ("string"), w158) -> (w159:string)
                n67 = GPIB Write(0:w156, 1:w159) -> ()  [unwired: 3 in, 2 out]
              }
              frame #1 {
                n68 = Wait (ms)(milliseconds to wait=u32 50) -> ()  [unwired: 1 out]
              }
              frame #2 {
                # "Measure the voltage"
                n69 = flat-sequence {
                  tunnel: w177 -> [w184]
                  tunnel: w176 -> [w182]
                  tunnel: w175 -> [w181]
                  tunnel: w174 -> [w183]
                  tunnel: [w186] -> w173
                  tunnel: [w185] -> w172
                  tunnel: w171 -> [w185]
                  tunnel: [w184] -> w170
                  tunnel: [w183] -> w169
                  tunnel: [w182] -> w168
                  tunnel: [w181] -> w167
                  tunnel: [w180] -> w166
                  tunnel: [w179] -> w165
                  tunnel: w173 -> [w192]
                  tunnel: w172 -> [w206]
                  tunnel: w170 -> [w205]
                  tunnel: w169 -> [w199]
                  tunnel: w168 -> [w198]
                  tunnel: w167 -> [w197]
                  tunnel: w166 -> [w191]
                  tunnel: w165 -> [w190]
                  frame #0 {
                    n70 = call "DC Basic Measure.vi"("Channel 2"=FALSE, "Voltmeter 2 Address"="8", "Channel 1"=TRUE, "Voltmeter 1 Address"=w184, "Period (s)"=w181, "Amplitude (A)"=w182) -> ("STD 1"=w179:dbl, "Resistance 1"=w178:dbl)  [unwired: 2 in, 2 out]
                    n71 = Multiply(x=w178, y=w183) -> (x*y=w186:dbl)
                    n72 = Multiply(x=w179, y=w183) -> (x*y=w180:dbl)
                  }
                  frame #1 {
                    n73 = Fract/Exp String To Number(string=w206) -> (number=w200:dbl)  [unwired: 3 in, 1 out]
                    n74 = Greater?(x=w192, y=w200) -> (0:w202:bool)
                    n75 = Less?(x=w200, y=100.0) -> (x < y?=w203:bool)
                    n76 = And(x=w202, y=w203) -> (x .and. y?=w201:bool)
                    n77 = case shown="True" w201 {
                      tunnel: w205 -> [_ w225]
                      tunnel: w200 -> [_ w224]
                      tunnel: w199 -> [w208 w215]
                      tunnel: w198 -> [_ w222]
                      tunnel: w197 -> [_ w221]
                      tunnel: [w209 w216] -> w195
                      tunnel: [w213 w219] -> w193
                      tunnel: [w212 w220] -> w194
                      tunnel: [w207 w214] -> w196
                      tunnel: w192 -> [w211 _]
                      tunnel: w191 -> [w213 _]
                      tunnel: w190 -> [w212 _]
                      frame False {
                        n78 = local read "Voltage Offset"() -> (w210:dbl)
                        n79 = Subtract(x=w211, y=w210) -> (x-y=w209:dbl)
                        n80 = Divide(x=w209, y=w208) -> (x/y=w207:dbl)
                      }
                      frame True {
                        n81 = flat-sequence {
                          tunnel: w225 -> [w227]
                          tunnel: w224 -> [w231]
                          tunnel: [w227] -> w223
                          tunnel: w215 -> [w242]
                          tunnel: w223 -> [w241]
                          tunnel: w222 -> [w240]
                          tunnel: w221 -> [w239]
                          tunnel: [w237] -> w218
                          tunnel: [w236] -> w219
                          tunnel: [w235] -> w220
                          frame #0 {
                            n82 = Multiply(x=w231, y=10.0) -> (x*y=w229:dbl)
                            n83 = Wait (ms)(milliseconds to wait=u32 100) -> ()  [unwired: 1 out]
                            n84 = Number To Exponential String(number=w229) -> (E-format string=w226:string)  [unwired: 3 in]
                            n85 = local write "2182A Range"(w226) -> ()
                            n86 = Concatenate Strings(":SENS:VOLT:DC:RANG " ("string"), w226) -> (w233:string)
                            n87 = GPIB Write(0:w227, 1:w233) -> ()  [unwired: 3 in, 2 out]
                          }
                          frame #1 {
                            n88 = call "DC Basic Measure.vi"("Channel 2"=FALSE, "Voltmeter 2 Address"="8", "Channel 1"=TRUE, "Voltmeter 1 Address"=w241, "Period (s)"=w239, "Amplitude (A)"=w240) -> ("STD 1"=w235:dbl, "Resistance 1"=w234:dbl)  [unwired: 2 in, 2 out]
                            n89 = Multiply(x=w234, y=w242) -> (x*y=w237:dbl)
                            n90 = Multiply(x=w235, y=w242) -> (x*y=w236:dbl)
                          }
                        }
                        n91 = local read "Voltage Offset"() -> (w217:dbl)
                        n92 = Subtract(x=w218, y=w217) -> (x-y=w216:dbl)
                        n93 = Divide(x=w216, y=w215) -> (x/y=w214:dbl)
                      }
                    }
                    n94 = local write "Voltage"(w195) -> ()
                    n95 = local write "Resistance"(w196) -> ()
                    n96 = local write "Resistance STD"(w194) -> ()
                    n97 = local write "Votlage STD"(w193) -> ()
                  }
                }
              }
              frame #3 {
                # "Resistance"
                # "Voltage"
                # "Current"
                # "Write data to output array"
                n98 = Wait (ms)(milliseconds to wait=u32 50) -> ()  [unwired: 1 out]
                n99 = local read "Current Now"() -> (w262:string)
                n100 = local read "Votlage STD"() -> (w253:dbl)
                n101 = local read "Voltage"() -> (w255:dbl)
                n102 = Fract/Exp String To Number(string=w262) -> (number=w252:dbl)  [unwired: 3 in, 1 out]
                n103 = Divide(x=w255, y=w252) -> (x/y=w254:dbl)
                n104 = Divide(x=w253, y=w252) -> (x/y=w251:dbl)
                n105 = local read "Data array"() -> (w260:dbl[][])
                n106 = Build Array(w252, w255, w253, w254, w251) -> (w261:dbl[])
                n107 = Insert Into Array(array=w260, new element=w261) -> (w259:dbl[][])  [unwired: 2 in]
                n108 = local write "Data array"(w259) -> ()
                n109 = Index Array(array=w259, index (col) #1=0 ("index (row)"), index (col) #2=1 ("index (row)"), index (col) #3=3 ("index (col)")) -> (element #1=w249:dbl[], element #2=w258:dbl[], element #3=w248:dbl[])  [unwired: 3 in]
                n110 = Bundle("Data array"=w249, "Data array"=w258) -> (w250:cluster{"Data array":dbl[], "Data array":dbl[]})  [unwired: 1 in]
                n111 = Bundle("Data array"=w249, "Data array"=w248) -> (w246:cluster{"Data array":dbl[], "Data array":dbl[]})  [unwired: 1 in]
                n112 = Build Array(w250, w246) -> (w245:T2)
                n113 = local write "I-V Plot"(w245) -> ()
              }
            }
          }
        }
      }
    }
    frame #4 {
      n114 = flat-sequence {
        tunnel: w264 -> [w266]
        tunnel: w265 -> [w269]
        frame #0 {
          # "Turn off the current source"
          n115 = Wait (ms)(milliseconds to wait=u32 1000) -> ()  [unwired: 1 out]
          n116 = GPIB Write(0:w266, 1:"OUTPUT OFF" ("data")) -> ()  [unwired: 3 in, 2 out]
        }
        frame #1 {
          n117 = case shown="False" w269 {
            frame False {
              n118 = invoke class="VI" method="FP.Close"() -> ()  [unwired: 3 in, 3 out]
            }
            frame True {
            }
          }
        }
      }
    }
  }
  "Current Samples" <- dbl[] [] ("array")
  "Data array" <- dbl[][] [] ("Data array")
